vi "app.vi"(2 "Read current":bool) -> ()   [LabVIEW 2019]
uses:
  <vilib>/Instr/_visa.llb/VISA Configure Serial Port (Instr).vi
  Program Files (x86)/National Instruments/LabVIEW 2019/examples/Instrument IO/Serial/support/Serial - Settings.ctl
panel:
  in  "ON":bool
  out "Current":string
  out "?":string
  out "?":string
  in  "Read voltage":bool
  out "Voltage":string
  in  "?":bool
  in  "?":bool
  in  "OK Volt":bool
  in  "Vset":dbl(knob) scale=0.0..30.0
  in  "OK Curr":bool
  in  "Iset":dbl(knob) scale=0.01..2.0
  in  "VISA Resource":refnum<visa-resource-name>="COM1"
  in  "Serial Settings (write)":T1={"baud rate"=9600, "data bits"=8, "parity"=enum."None", "stop bits"=10, "flow control"=0} {"flow control" items=["None"=0, "XON/XOFF"=1, "RTS/CTS"=2, "DTR/DSR"=4]; "stop bits" items=["1.0"=10, "1.5"=15, "2.0"=20]; "data bits" min=5 max=8 step=1; "baud rate" items=["75"=75, "110"=110, "134"=134, "150"=150, "300"=300, "600"=600, "1200"=1200, "1800"=1800, "2400"=2400, "4800"=4800, "7200"=7200, "9600"=9600, "14400"=14400, "19200"=19200, "28800"=28800, "38400"=38400, "56000"=56000, "57600"=57600, "115200"=115200, "128000"=128000, "230400"=230400]}
  # "OFF"
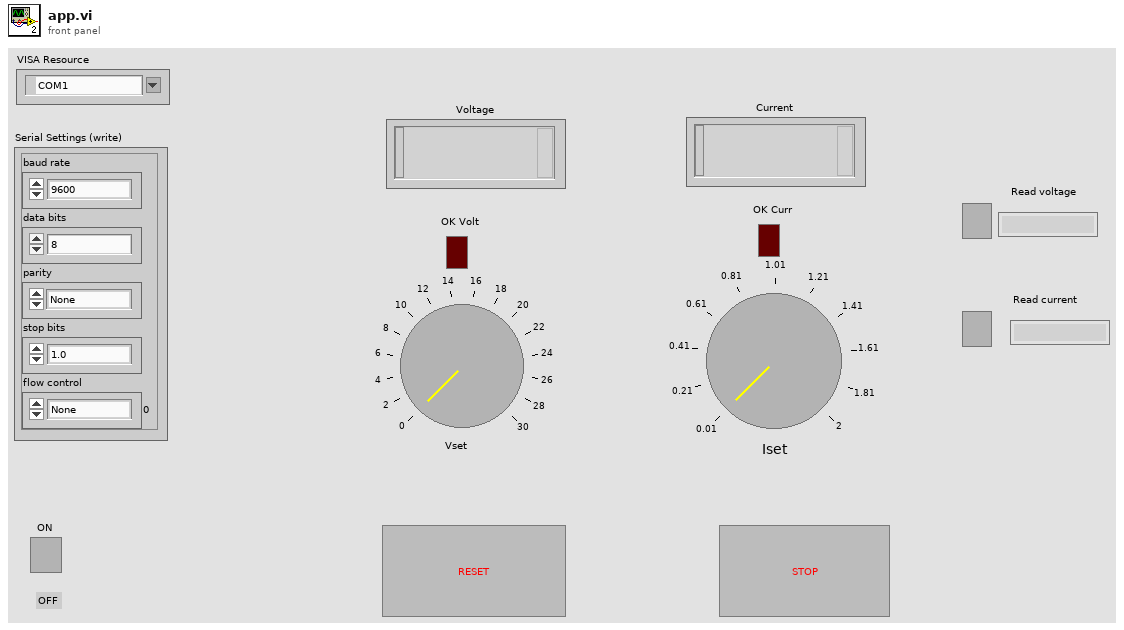
[diagram p1: front panel]
types:
  T1 = typedef "Serial - Settings.ctl" = cluster{"baud rate":u32, "data bits":u16, "parity":enum16{"None", "Odd", "Even", "Mark", "Space"}, "stop bits":u16, "flow control":u16}
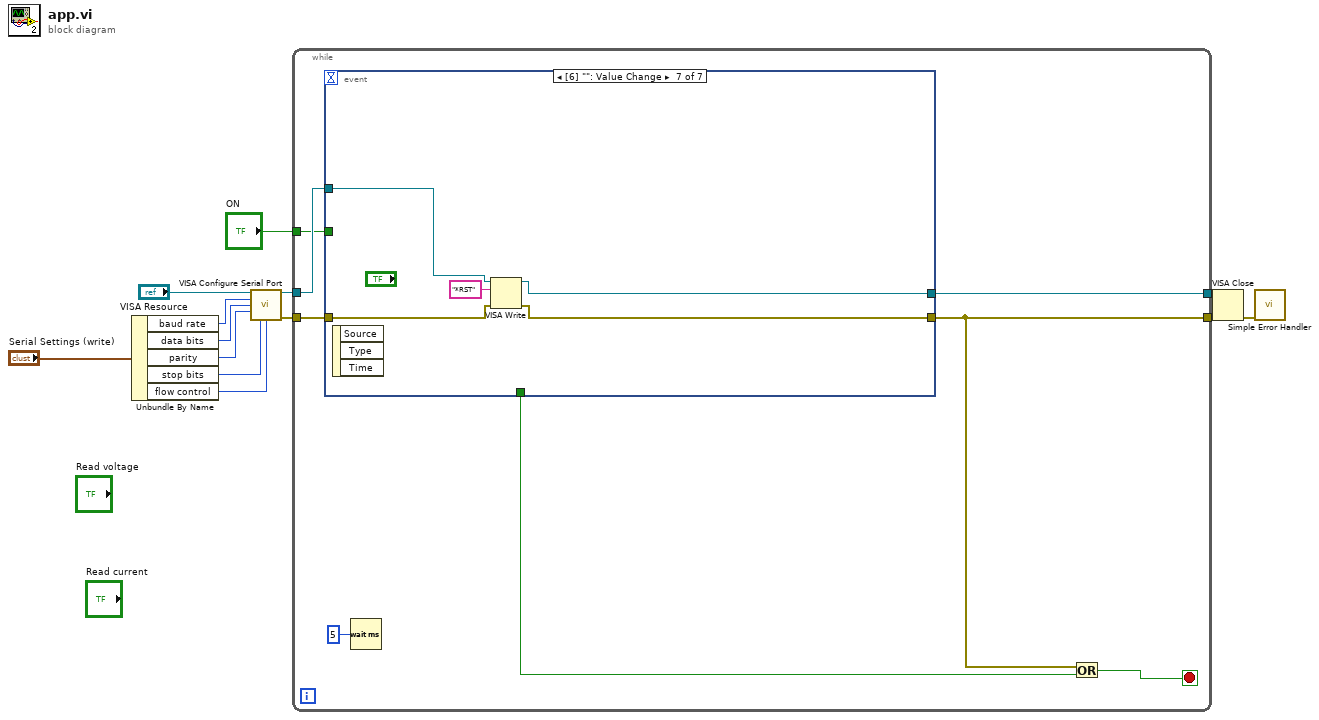
[diagram p0: block diagram]
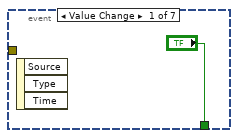
[diagram p2: hidden frame]
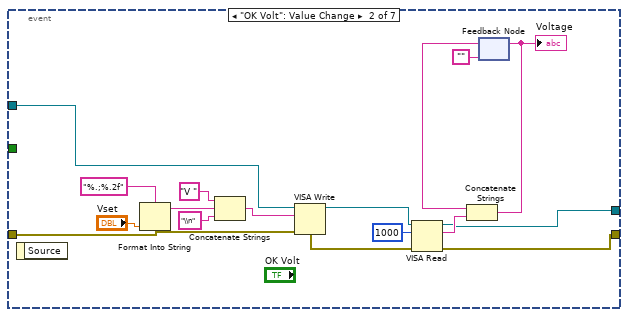
[diagram p3: hidden frame]
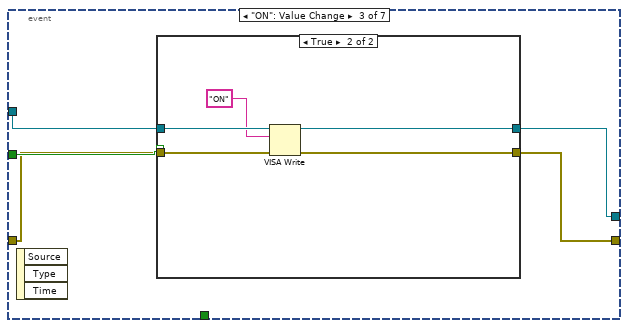
[diagram p4: hidden frame]
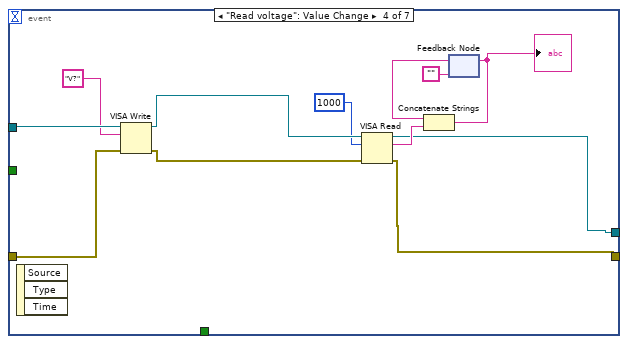
[diagram p6: hidden frame]
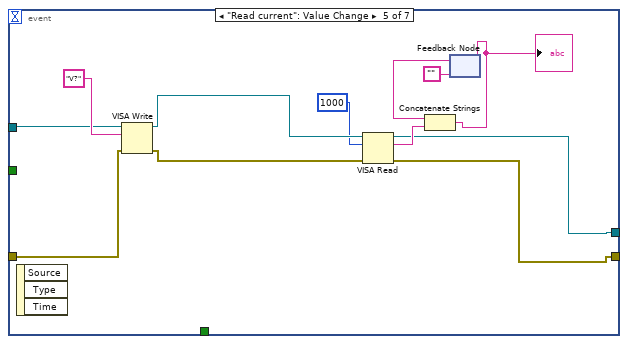
[diagram p7: hidden frame]
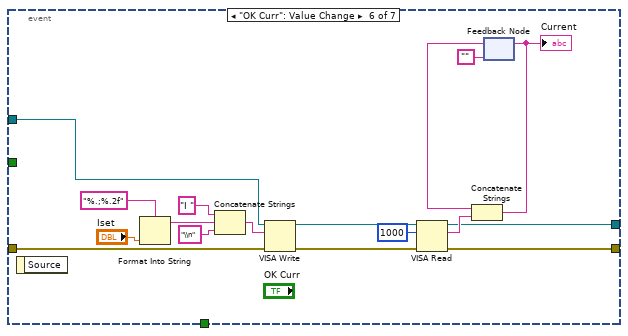
[diagram p8: hidden frame]
diagram:
  n1 = Unbundle By Name("Serial Settings (write)") -> ("baud rate"=w10:u32, "data bits"=w9:u16, "parity"=w8:enum16{"None", "Odd", "Even", "Mark", "Space"}, "stop bits"=w7:u16, "flow control"=w6:u16)
  n2 = call-poly "VISA Configure Serial Port"("VISA resource name"="VISA Resource", "baud rate (9600)"=w10, "data bits (8)"=w9, "parity (0:none)"=w8, "stop bits (10: 1 bit)"=w7, "flow control (0:none)"=w6) -> ("VISA resource name out"=w5:refnum<visa-resource-name>, "error out"=w4:errorcluster)  [unwired: 3 in, 5 out]
  n3 = while {
    tunnel: w5 -> [w21]
    tunnel: w4 -> [w20]
    tunnel: [w15] -> w3
    tunnel: [w19] -> w2
    tunnel: "ON" -> [w14]
    stop <- w17 stop-if-true
    n4 = event shown="[6] \"\": Value Change" {
      selector: _ -> [_ _ _ _ _ _ _]
      dyn-events: _ -> [_ _ _ _ _ _ _]
      timeout: _ -> [_ _ _ _ _ _ _]
      tunnel: w21 -> [_ w32 w43 w61 w67 w84 w94]
      tunnel: w20 -> [_ w33 w42 w60 w66 w83 w93]
      tunnel: [_ w24 w40 w53 w65 _ w91] -> w15
      tunnel: [_ w25 w41 w52 w64 w76 w92] -> w19
      tunnel: ["?" _ _ _ _ _ _] -> w16
      tunnel: [_ _ _ _ _ w75 _] -> _
      tunnel: w14 -> [_ _ w44 _ _ _ _]
      event Value Change {
        n5 = event-data() -> ()  [unwired: 1 in, 3 out]
      }
      event "OK Volt": Value Change {
        n6 = event-data() -> ()  [unwired: 1 in, 1 out]
        n7 = Format Into String(format string="%.;%.2f", "Vset") -> (resulting string=w36:string)  [unwired: 2 in, 1 out]
        n8 = Concatenate Strings("V " ("string"), w36, "\\n" ("string")) -> (w34:string)
        n9 = VISA Write(VISA resource name=w32, write buffer=w34, error in (no error)=w33) -> (VISA resource name out=w27:refnum<visa-resource-name>, error out=w26:errorcluster)  [unwired: 1 out]
        n10 = VISA Read(VISA resource name=w27, byte count=u32 1000, error in (no error)=w26) -> (VISA resource name out=w25:refnum<visa-resource-name>, read buffer=w31:string, error out=w24:errorcluster)  [unwired: 1 out]
        n11 = feedback #1("") -> (w30:string)
        n12 = Concatenate Strings(w30, w31) -> (w29:string)
        "Voltage" <- w29
        n13 = feedback-in #1(w29) -> ()
      }
      event "ON": Value Change {
        n14 = event-data() -> ()  [unwired: 1 in, 3 out]
        n15 = case shown="True" w44 {
          tunnel: w43 -> [_ w49]
          tunnel: w42 -> [_ w48]
          tunnel: [_ w46] -> w41
          tunnel: [_ w45] -> w40
          frame False {
          }
          frame True {
            n16 = VISA Write(VISA resource name=w49, write buffer="ON", error in (no error)=w48) -> (VISA resource name out=w46:refnum<visa-resource-name>, error out=w45:errorcluster)  [unwired: 1 out]
          }
        }
      }
      event "Read voltage": Value Change {
        n17 = event-data() -> ()  [unwired: 1 in, 3 out]
        n18 = VISA Write(VISA resource name=w61, write buffer="V?", error in (no error)=w60) -> (VISA resource name out=w55:refnum<visa-resource-name>, error out=w54:errorcluster)  [unwired: 1 out]
        n19 = VISA Read(VISA resource name=w55, byte count=u32 1000, error in (no error)=w54) -> (VISA resource name out=w52:refnum<visa-resource-name>, read buffer=w58:string, error out=w53:errorcluster)  [unwired: 1 out]
        n20 = feedback #2("") -> (w57:string)
        n21 = Concatenate Strings(w57, w58) -> (w51:string)
        "?" <- w51
        n22 = feedback-in #2(w51) -> ()
      }
      event "Read current": Value Change {
        n23 = event-data() -> ()  [unwired: 1 in, 3 out]
        n24 = VISA Write(VISA resource name=w67, write buffer="V?", error in (no error)=w66) -> (VISA resource name out=w72:refnum<visa-resource-name>, error out=w73:errorcluster)  [unwired: 1 out]
        n25 = VISA Read(VISA resource name=w72, byte count=u32 1000, error in (no error)=w73) -> (VISA resource name out=w64:refnum<visa-resource-name>, read buffer=w70:string, error out=w65:errorcluster)  [unwired: 1 out]
        n26 = feedback #3("") -> (w71:string)
        n27 = Concatenate Strings(w71, w70) -> (w63:string)
        "?" <- w63
        n28 = feedback-in #3(w63) -> ()
      }
      event "OK Curr": Value Change {
        n29 = event-data() -> ()  [unwired: 1 in, 1 out]
        n30 = Format Into String(format string="%.;%.2f", "Iset") -> (resulting string=w87:string)  [unwired: 2 in, 1 out]
        n31 = Concatenate Strings("I " ("string"), w87, "\\n" ("string")) -> (w85:string)
        n32 = VISA Write(VISA resource name=w84, write buffer=w85, error in (no error)=w83) -> (VISA resource name out=w78:refnum<visa-resource-name>, error out=w77:errorcluster)  [unwired: 1 out]
        n33 = VISA Read(VISA resource name=w78, byte count=u32 1000, error in (no error)=w77) -> (VISA resource name out=w76:refnum<visa-resource-name>, read buffer=w82:string, error out=w75:errorcluster)  [unwired: 1 out]
        n34 = feedback #4("") -> (w81:string)
        n35 = Concatenate Strings(w81, w82) -> (w80:string)
        "Current" <- w80
        n36 = feedback-in #4(w80) -> ()
      }
      event Value Change {
        n37 = event-data() -> ()  [unwired: 1 in, 3 out]
        n38 = VISA Write(VISA resource name=w94, write buffer="*RST", error in (no error)=w93) -> (VISA resource name out=w92:refnum<visa-resource-name>, error out=w91:errorcluster)  [unwired: 1 out]
      }
    }
    n39 = Wait (ms)(milliseconds to wait=u32 5) -> ()  [unwired: 1 out]
    n40 = Or(x=w15, y=w16) -> (x .or. y?=w17:bool)
  }
  n41 = VISA Close(VISA resource name=w2, error in (no error)=w3) -> (error out=w13:errorcluster)
  n42 = call <vilib>:"Simple Error Handler.vi"("error in (no error)"=w13) -> ()  [unwired: 1 in, 8 out]
